vi "Generic Device VI Tester.vi"   [LabVIEW 2011]
uses:
  Private/Device/Device.lvlib
types:
  T1 = typedef "LVH-LINX.lvlib/Device.lvlib/LINX Device Config.ctl" = cluster{"Interface":T2, "COM Port":refnum<visa-resource-name>, "TCP Configuration":T3, "Device ID":u8, "Device Name":string, "Device Family":T4}
  T2 = typedef "LVH-LINX.lvlib/Interface.ctl" = enum16{"Serial", "TCP"}
  T3 = typedef "LVH-LINX.lvlib/Device.lvlib/TCP Config.ctl" = cluster{"IP Address":string, "Port":dbl}
  T4 = typedef "LVH-LINX.lvlib/Device Family.ctl" = enum8{"National Instruments", "Digilent", "Arduino"}
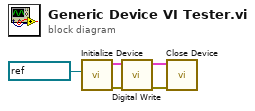
[diagram p0: block diagram]
diagram:
  n1 = call "Initialize Device.vi"("COM Port"=refnum<visa-resource-name> "COM5") -> ("Error Out"=w1:errorcluster, "LINX Device Config"=w4:T1)  [unwired: 9 in]
  n2 = call "Digital Write.vi"("Error In"=w1, "LINX Device Config"=w4) -> ("Error Out"=w2:errorcluster, "LINX Device Config"=w3:T1)  [unwired: 8 in]
  n3 = call "Close Device.vi"("Error In"=w2, "LINX Device Config"=w3) -> ()  [unwired: 8 in, 2 out]
